vi "Clean.vi"(8 "error in (no error)":errorcluster, 11 "Task in":refnum<class "Task.lvclass">) -> (0 "error out":errorcluster, 3 "Task out":refnum<class "Task.lvclass">)   [LabVIEW 2017, in "Task Interface.lvlib" / "Task.lvclass"]
uses:
  Task.lvclass
  Task.lvclass/Task.ctl
  <vilib>/AppBuilder/AB_API_Simple/NI_App_Builder_API.lvlib
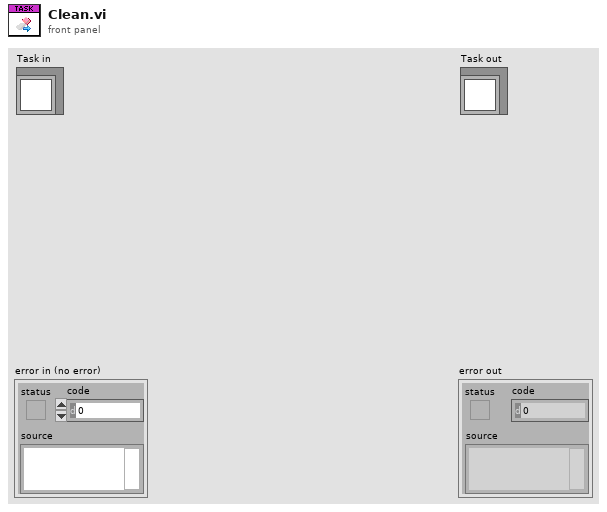
[diagram p1: front panel]
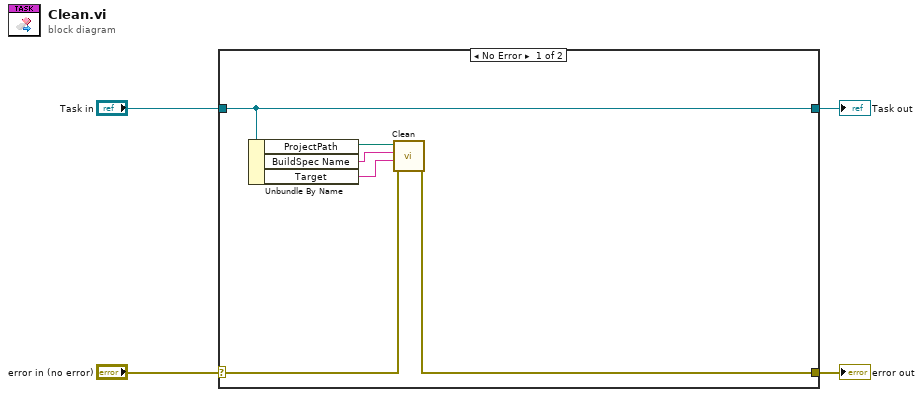
[diagram p0: block diagram]
diagram:
  n1 = case shown="No Error" "error in (no error)" {
    selector: "error in (no error)" -> [w6 w12]
    tunnel: [w5 w12] -> w3
    tunnel: [w10 w11] -> w1
    tunnel: "Task in" -> [w10 w11]
    frame No Error {
      n2 = Unbundle By Name(w10) -> ("ProjectPath"=w9:path, "BuildSpec Name"=w8:string, "Target"=w7:string)
      n3 = call <vilib>:"Clean.vi"("error in (no error)"=w6, "Name of target (My Computer)"=w7, "Name of build specification (if empty: clean all)"=w8, "Path to project"=w9) -> ("error out"=w5:errorcluster)  [unwired: 7 in]
    }
    frame Error {
    }
  }
  "error out" <- w3
  "Task out" <- w1
